vi "sleep_deprivation.vi"(2 "Deprivation\nparameters":T1={"Frame Row"=0, "Kstd"=40.0, "# Images for\nsleep detection"=10, "Kmean"=1.5, "Start time of sleep detection (images):"=1000, 0, "Length (images)"=3600, "# TTL"=10000, "by x images after first detection"=0, "Between TTL pulses"=0, "\nby x detections"=9, "# Total immobility\n detections"=0.0, "max # adjacent\nTTL"=0.0, "TTL x start\ntime deprivation\n"=0.0, "Max #\nadjacent TTL"=10000, " Ca2+\nmode"=0} {"?" items=["1", "2", "3", "4"]; "Frame Row" items=["1", "2", "3", "4"]}, 3 "Input \nparameters":T3={"Frame rate (ms)"=2000, "Worm strain"="N2", "Time t"=0, "State"=enum."Image acquisition", "Time elapsed"=0.0, "Max_num_runs"=100000, "#TTL"=0, "Time of start TTL"=100000, "ImSub Value"=0, "Time of last TTL"=0, "Number of Columns"=2, "Number of Rows"=2, "# AdjacentTTL"=0, "Sleep deprivation status"="", "Sleep Detection"=FALSE, "# Sleep detections"=0, "Time of first sleep detection"=0, "Time max # adjacent TTL"=0, "Image t-1"=[], "Image t"=[]} {"Number of Rows" items=["1"=1, "2"=2, "3"=3, "4"=4]; "Number of Columns" items=["1"=1, "2"=2, "3"=3, "4"=4]}, 4 "#TTL change\nmode":dbl=10000.0, 5 "Second deprivation method":T4={"lines"="Dev1/port2/line7", "Pause Time (ms)"=0, "Pulse Length (ms)"=300, "Number of Pulses"=1}, 6 "First deprivation method":T4={"lines"="Dev1/port2/line6", "Pause Time (ms)"=0, "Pulse Length (ms)"=15, "Number of Pulses"=1}) -> (1 "Output \nparameters":T3={"Frame rate (ms)"=2000, "Worm strain"="N2", "Time t"=0, "State"=enum."Image acquisition", "Time elapsed"=0.0, "Max_num_runs"=100000, "#TTL"=0, "Time of start TTL"=100000, "ImSub Value"=0, "Time of last TTL"=0, "Number of Columns"=2, "Number of Rows"=2, "# AdjacentTTL"=0, "Sleep deprivation status"="", "Sleep Detection"=FALSE, "# Sleep detections"=0, "Time of first sleep detection"=0, "Time max # adjacent TTL"=0, "Image t-1"=[], "Image t"=[]} {"Number of Rows" items=["1"=1, "2"=2, "3"=3, "4"=4]; "Number of Columns" items=["1"=1, "2"=2, "3"=3, "4"=4]})   [LabVIEW 2011]
uses:
  state.ctl
panel:
  # "Sleep deprivation settings"
  # "Select deprivation animal"
  # "Row"
  # "Column"
  # "Sleep detection parameters"
  # "Sleep deprivation parameters"
  # "Delay deprivation start:"
  # "Pause deprivation (images):"
  # "Stop deprivation after:"
  # "Line 7 LED"
  # "Line 6 Tap Magnet"
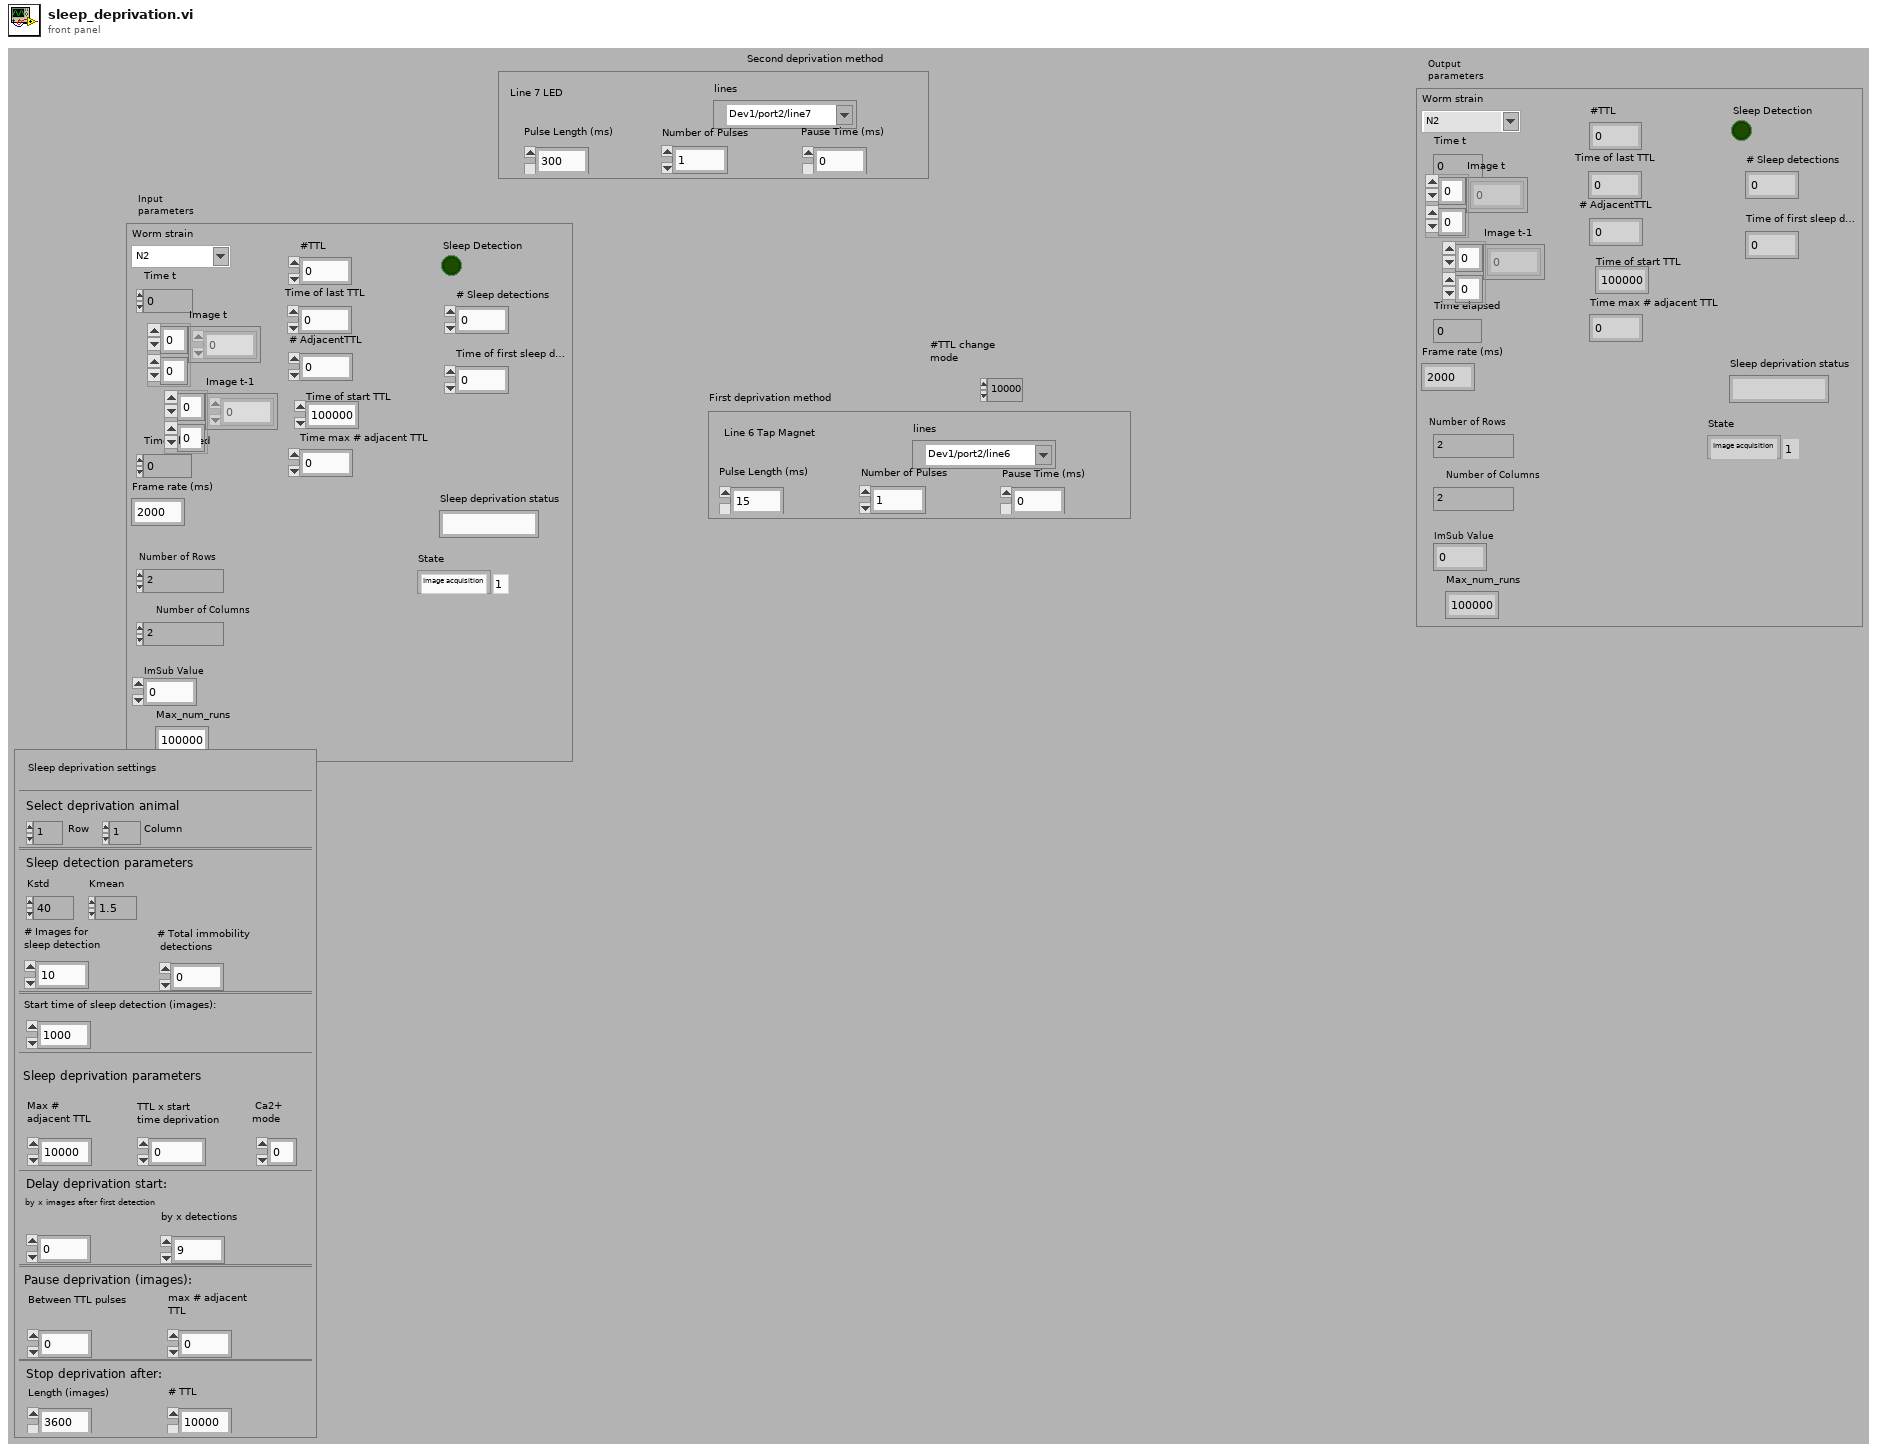
[diagram p1: front panel]
types:
  T1 = cluster{"Frame Row":u32, "Kstd":dbl, "# Images for\nsleep detection":i32, "Kmean":dbl, "Start time of sleep detection (images):":i32, u32, "Length (images)":i32, "# TTL":i32, "by x images after first detection":i32, "Between TTL pulses":i32, "\nby x detections":i32, "# Total immobility\n detections":dbl, "max # adjacent\nTTL":dbl, "TTL x start\ntime deprivation\n":dbl, "Max #\nadjacent TTL":i32, " Ca2+\nmode":i32}
  T2 = typedef "state.ctl" = enum16{"Initialize measurement", "Image acquisition", "Image processing", "Sleep detection", "Control TTL protocol ", "Sleep deprivation", "Update image & exit condition", "Wait "}
  T3 = cluster{"Frame rate (ms)":u32, "Worm strain":string, "Time t":i32, "State":T2, "Time elapsed":dbl, "Max_num_runs":i32, "#TTL":i32, "Time of start TTL":i32, "ImSub Value":i32, "Time of last TTL":i32, "Number of Columns":u32, "Number of Rows":u32, "# AdjacentTTL":i32, "Sleep deprivation status":string, "Sleep Detection":bool, "# Sleep detections":i32, "Time of first sleep detection":i32, "Time max # adjacent TTL":i32, "Image t-1":i32[][], "Image t":i32[][]}
  T4 = cluster{"lines":tag, "Pause Time (ms)":u32, "Pulse Length (ms)":u32, "Number of Pulses":i32}
  T5 = cluster{"Frame rate (ms)":u32, "Worm strain":string, "Time t":i32, "State":T2, "Time elapsed":dbl, "Max_num_runs":i32, "#TTL":i32, "SD start referenceL":i32, "ImSub Value":i32, "Time of last TTL":i32, "Number of Columns":u32, "Number of Rows":u32, "# AdjacentTTL":i32, "Sleep deprivation status":string, "Sleep Detection":bool, "# Sleep detections":i32, "Time of first sleep detection":i32, "Time max # adjacent TTL":i32, "Image t-1":i32[][], "Image t":i32[][]}
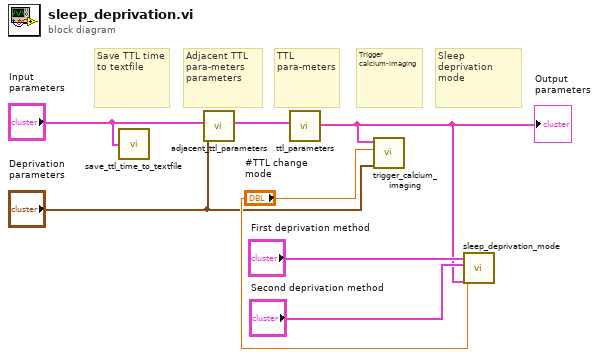
[diagram p0: block diagram]
diagram:
  # "TTL \npara-meters"
  # "Sleep\ndeprivation\nmode"
  # "Trigger\ncalcium-imaging"
  # "Adjacent TTL para-meters \nparameters"
  # "Save TTL time\nto textfile"
  n1 = call "save_ttl_time_to_textfile.vi"("Input \nparameters"="Input \nparameters") -> ()  [unwired: 5 in]
  n2 = call "adjacent_ttl_parameters.vi"("Deprivation\nparameters"="Deprivation\nparameters", "Input \nparameters"="Input \nparameters") -> ("Output \nparameters"=w3:T3)  [unwired: 9 in]
  n3 = call "ttl_parameters.vi"("Input \nparameters"=w3) -> ("Output \nparameters"=w2:T5)  [unwired: 5 in]
  "Output \nparameters" <- w2
  n4 = call "trigger_calcium_imaging.vi"("Input \nparameters"=w2, "#TTL change\nmode"="#TTL change\nmode", "Deprivation\nparameters"="Deprivation\nparameters") -> ()  [unwired: 8 in]
  n5 = call "sleep_deprivation_mode.vi"("Input \nparameters"=w2, "#TTL change\nmode"="#TTL change\nmode", "Second \nDeprivation Method"="Second deprivation method", "First \nDeprivation Method"="First deprivation method") -> ()  [unwired: 8 in]
